vi "Begin.vi"(8 "error in (no error)":errorcluster, 10 "variant in":variant, 11 "Robot in":refnum<class "Robot.lvclass">) -> (0 "error out":errorcluster, 3 "Robot out":refnum<class "Robot.lvclass">)   [LabVIEW 2019, in "Robot.lvlib" / "Robot.lvclass"]
uses:
  Robot.lvclass
  Robot.lvclass/Robot.ctl
  51b72ce7-4d66-448a-8d72-8faa07e8051f.vi
  78479825-048e-4f98-99aa-7665ebc65d47.vi
  <vilib>/Utility/error.llb/Trim Whitespace.vi
  <vilib>/Utility/error.llb/Error Cluster From Error Code.vi
panel:
  out "found 2":bool
  out "found":bool
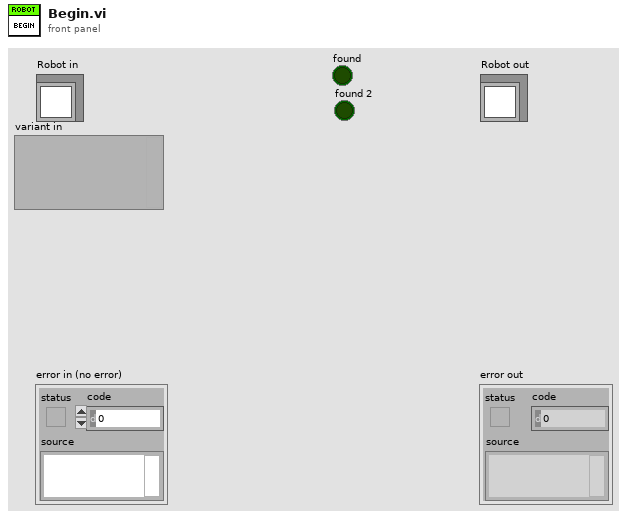
[diagram p1: front panel]
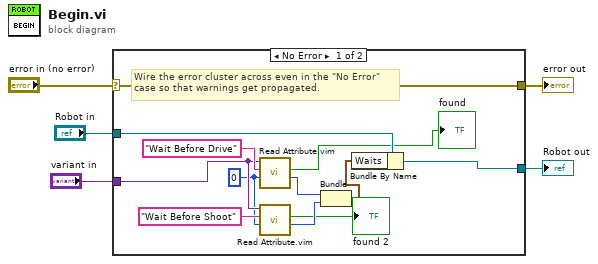
[diagram p0: block diagram]
diagram:
  n1 = case shown="No Error" "error in (no error)" {
    selector: "error in (no error)" -> [w17 w19]
    tunnel: [w17 w19] -> w4
    tunnel: [w11 w18] -> w2
    tunnel: "Robot in" -> [w12 w18]
    tunnel: "variant in" -> [w15 _]
    frame No Error {
      w13 = 0
      # "Wire the error cluster across even in the \"No Error\"\ncase so that warnings get propagated."
      n2 = call "Read Attribute.vim"("default value (data type)"=w13, "name"="Wait Before Drive", "variant in"=w15) -> ("value"=w10:i32, "found"=→"found":bool)  [unwired: 5 in, 2 out]
      n3 = call "Read Attribute.vim"("default value (data type)"=w13, "name"="Wait Before Shoot", "variant in"=w15) -> ("value"=w9:i32, "found"=→"found 2":bool)  [unwired: 5 in, 2 out]
      n4 = Bundle("value"=w10, "value"=w9) -> (w8:cluster{"value":i32, "value":i32})  [unwired: 1 in]
      n5 = Bundle By Name(cluster=w12, "Waits"=w8) -> (w11:refnum<class "Robot.lvclass">)
    }
    frame Error {
    }
  }
  "error out" <- w4
  "Robot out" <- w2
